vi "GetGyroAngle.vi"(8 "error in":errorcluster) -> (0 "error out":errorcluster, 3 "Angle":dbl)   [LabVIEW 2016]
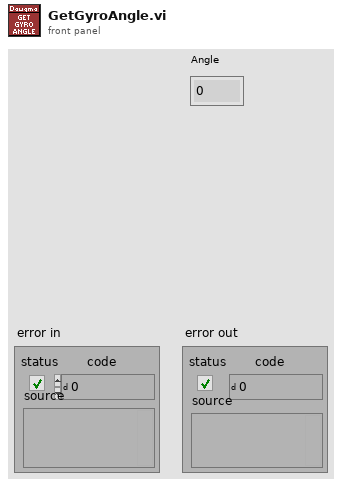
[diagram p1: front panel]
types:
  T1 = cluster{"Yaw":dbl, "Roll":dbl, "Pitch":dbl, "Heading":dbl, "Fused Heading":dbl}
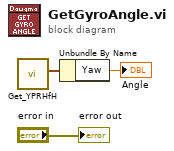
[diagram p0: block diagram]
diagram:
  n1 = call <vilib>:"Get_YPRHfH.vi"() -> ("YRPHfH"=w2:T1)  [unwired: 11 in]
  n2 = Unbundle By Name(w2) -> ("Yaw"=→"Angle":dbl)
  "error out" <- "error in"
